vi "电导率电极校准.vi"() -> ()   [LabVIEW 2016, in "斯坦道多参数.lvlib"]
uses:
  <vilib>/Utility/miscctls.llb/LVPointTypeDef.ctl
  <vilib>/Analysis/NI_AALBase.lvlib
panel:
  out "通讯状态":string
  out "盐度":dbl caption="盐度测量值" format="%#.2f"
  out "温度":dbl format="%#.2f"
  out "当前信号值":dbl caption="信号值" format="%#.2f"
  in  "校准停止":bool
  in  "校准启动":bool
  out "波形图表":sgl(graph) caption="历史曲线"
  out "第二点校准值":dbl
  out "第一点校准值":dbl
  in  "校准模式":enum16{"两点校准", "单点校准"}(ring)=enum."单点校准"
  out "提示":string
  out "最小值":sgl format="%#.2f"
  out "最大值":sgl format="%#.2f"
  out "mean":dbl caption="均值" format="%#.2f"
  out "standard deviation":dbl caption="标准差" format="%#.2f"
  out "变异系数":dbl format="%#.6f"
  out "标液2":dbl
  out "标液1":dbl
  out "当前读取值":dbl caption="测量值" format="%#.2f"
  out "电极系数":dbl format="%#.6f"
  out "偏移值补偿":dbl format="%#.2f"
  out "温度补偿系数":dbl caption="温度系数" format="%#.6f"
  # "电导率电极设定"
  # "ppt"
  # "请选择校准模式:"
  # "℃"
  # "uS/cm"
  # "uS/cm"
  # "cm"
  # "-1"
  # "uS/cm"
  # "%"
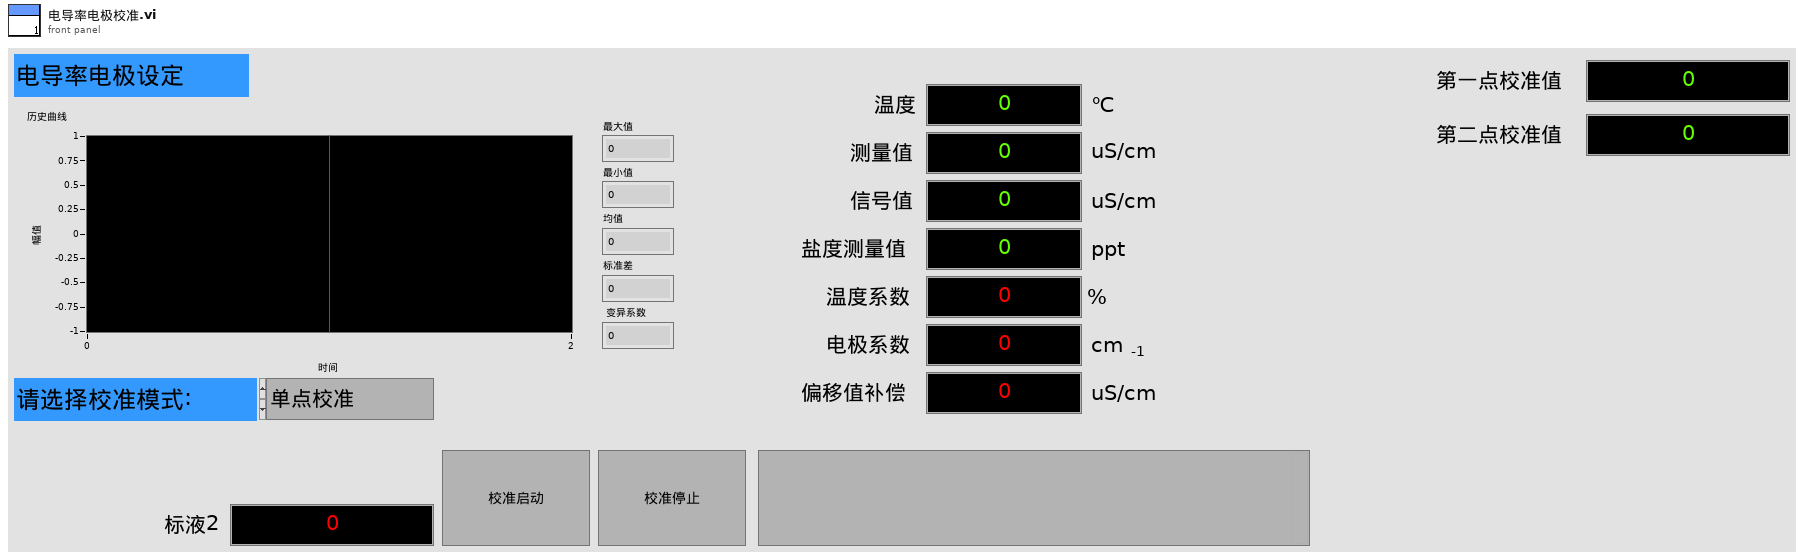
[diagram p1: front panel]
types:
  T1 = typedef "斯坦道多参数.lvlib/校准步骤.ctl" = enum16{"待机", "放置第一点标液", "第一点校准启动", "第一点校准写入", "第一点校准失败", "放置第二点标液", "第二点校准启动", "第二点校准写入", "第二点校准失败", "放置第三点标液", "第三点校准启动", "第三点校准写入", "第三点校准失败", "校准结果写入", "校准结束"}
  T2 = typedef "LVPointTypeDef.ctl" = cluster{"Horizontal":i16, "Vertical":i16}
  T3 = cluster{"电极状态标志":u16, "电极型号标志":u16, "电导率测量值":sgl, "温度测量值":sgl, "电导率信号值":sgl, "温度信号值":sgl, "温度补偿系数":sgl, "电导率偏移修正值":sgl, "温度偏移修正值":sgl, "手动温度补偿值":sgl, "电导率电极零点":sgl, "电导率电极斜率":sgl, "命令滤波设定":u16, "温度模式":enum16{"ATC", "MTC"}, "生产批次":u16, "电极序号":u16, "串口地址":u16, "串口波特率":enum16{"9600", "19200", "115200"}, "串口校验位":enum16{"NONE", "ODD", "EVEN"}, "串口停止位":enum16{"1bit", "2bit"}, "第一点标准值":sgl, "第二点标准值":sgl}
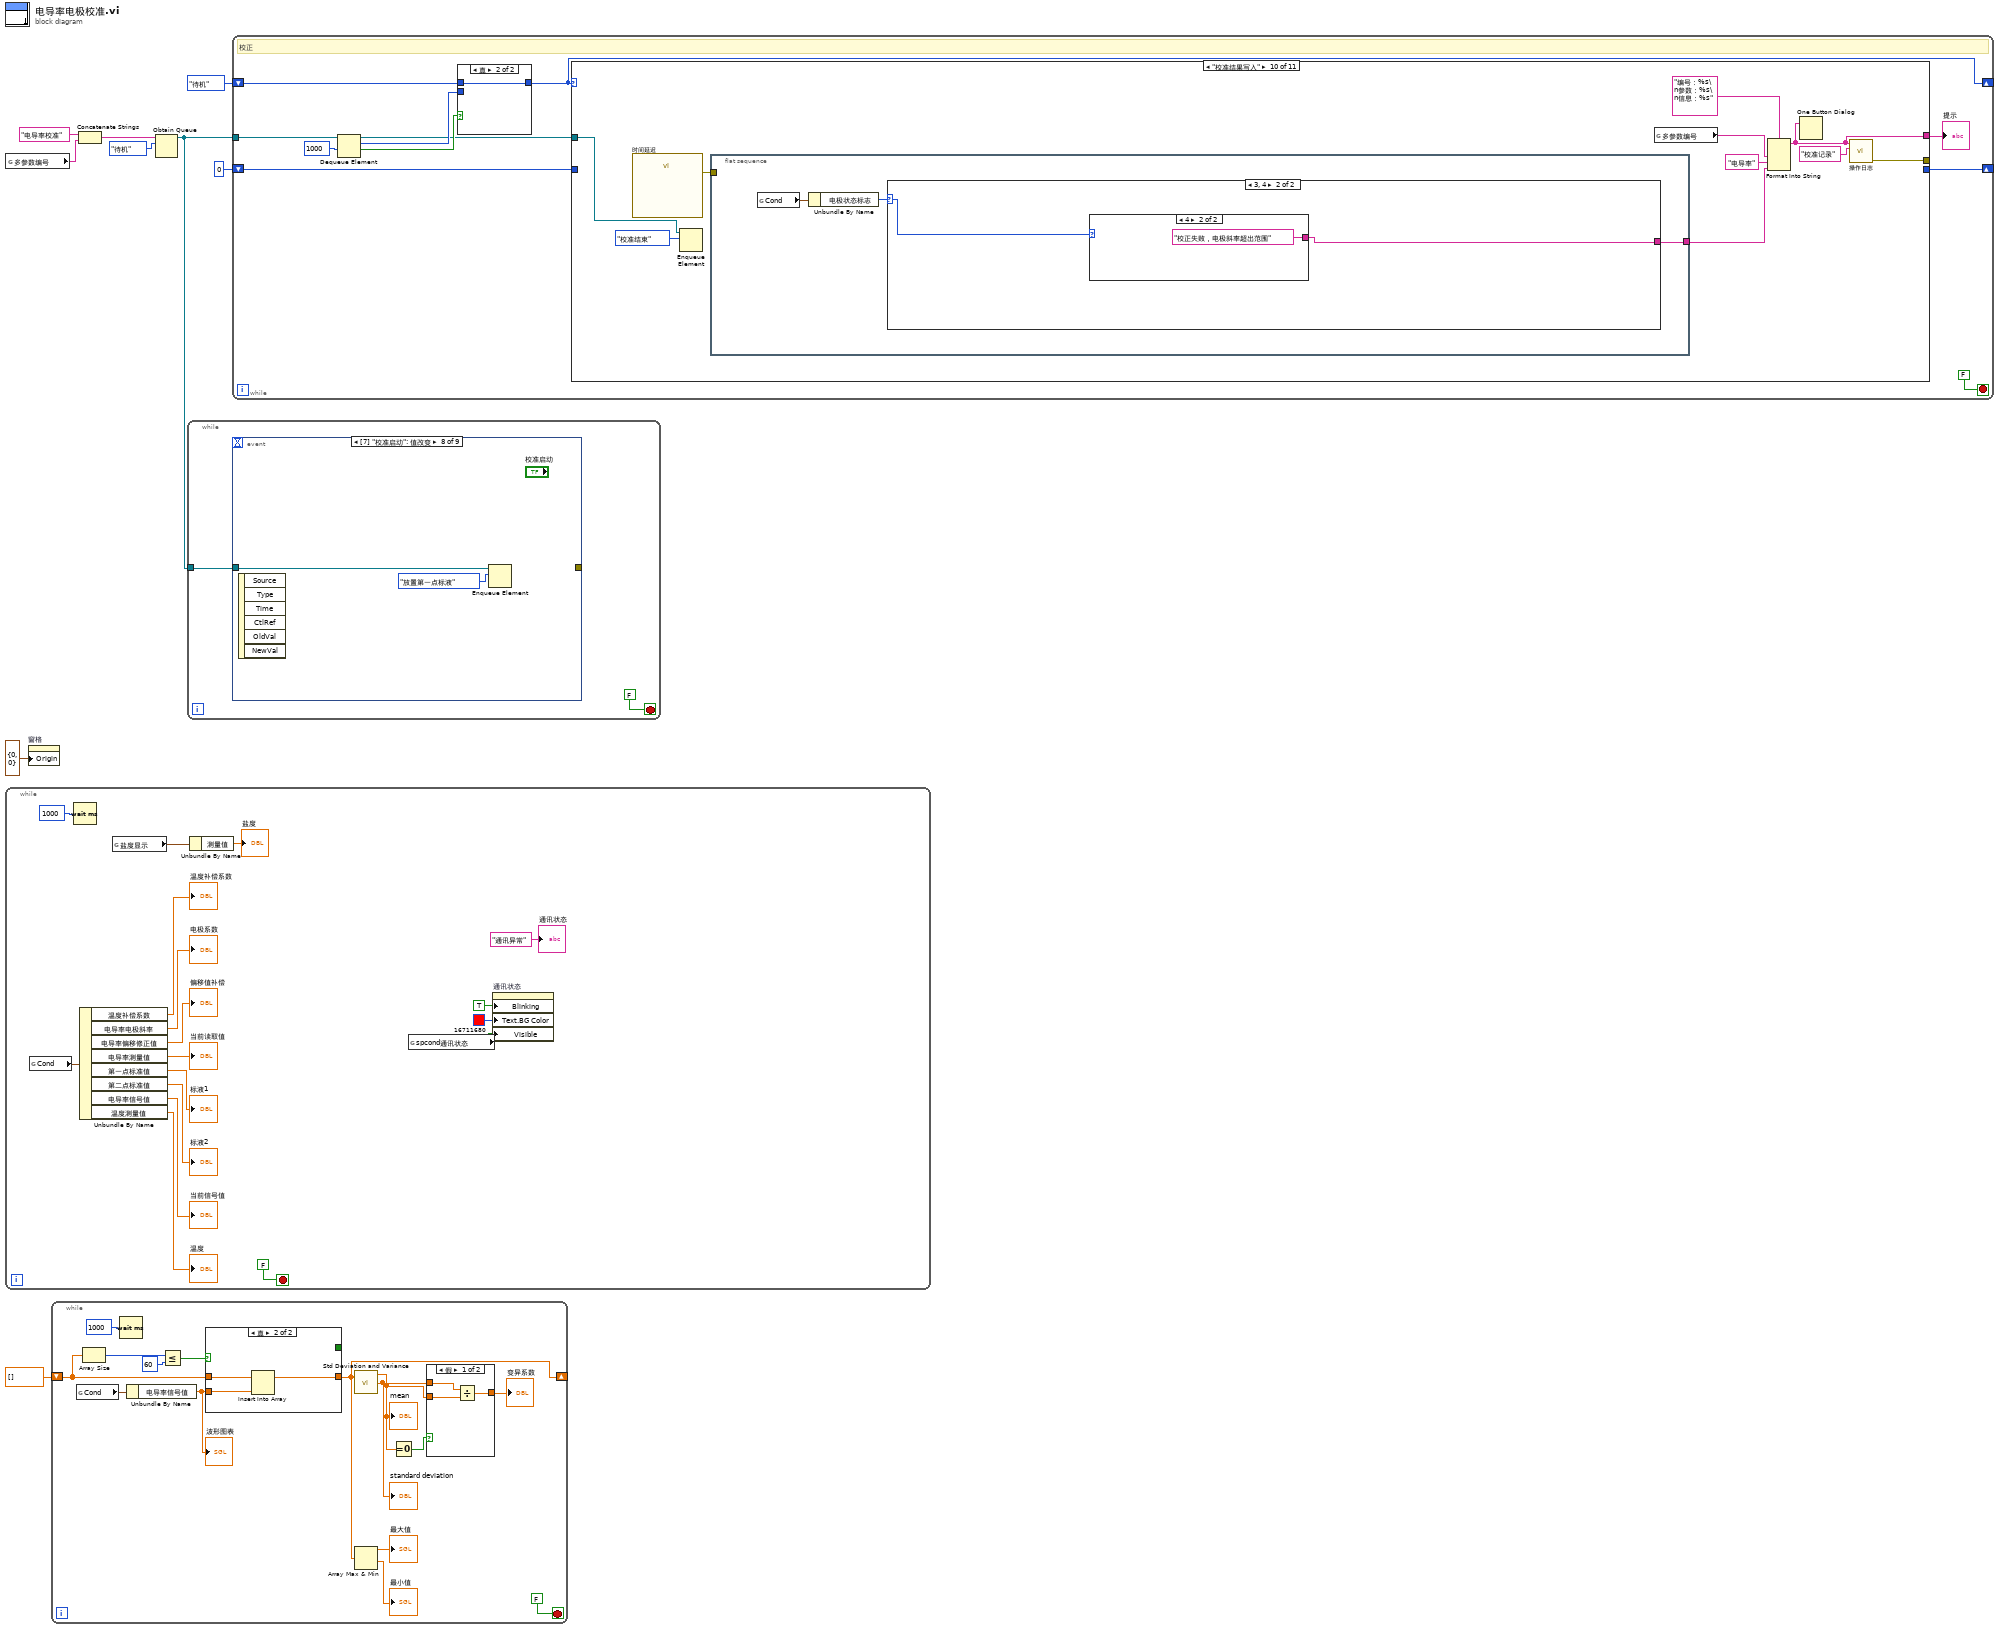
[diagram p0: block diagram]
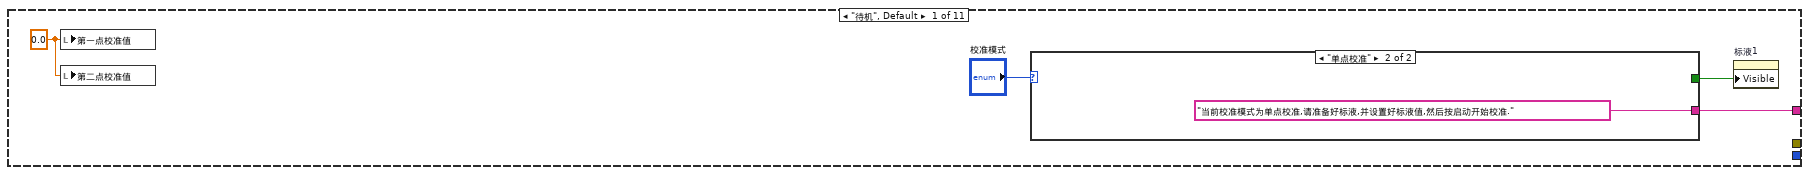
[diagram p3: hidden frame]
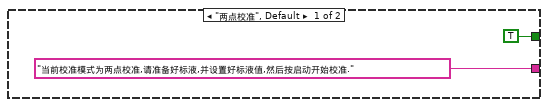
[diagram p4: hidden frame]
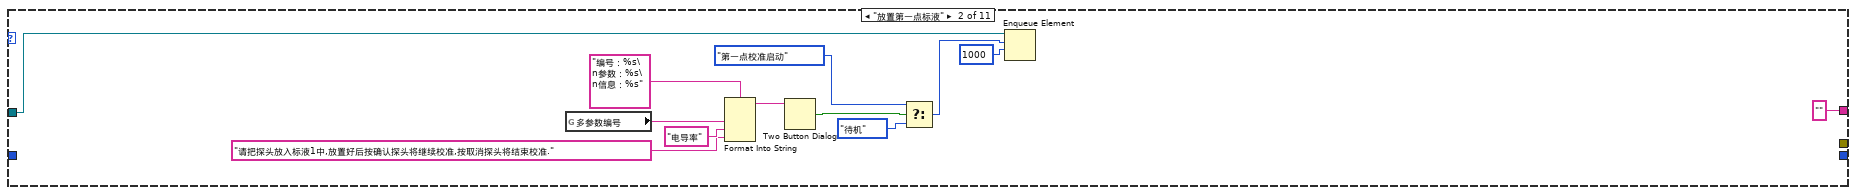
[diagram p5: hidden frame]
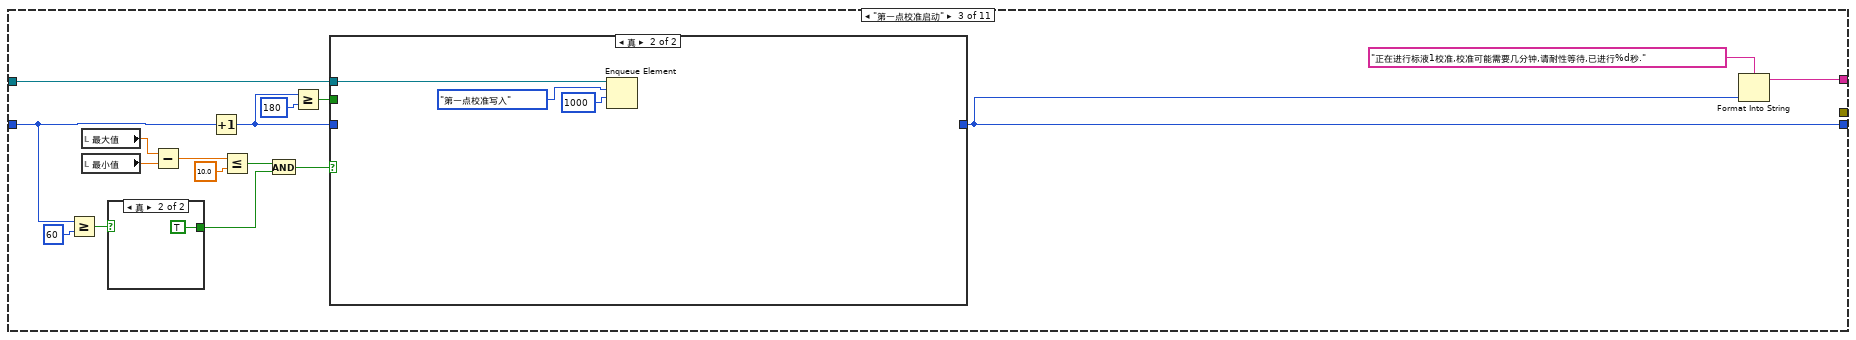
[diagram p6: hidden frame]
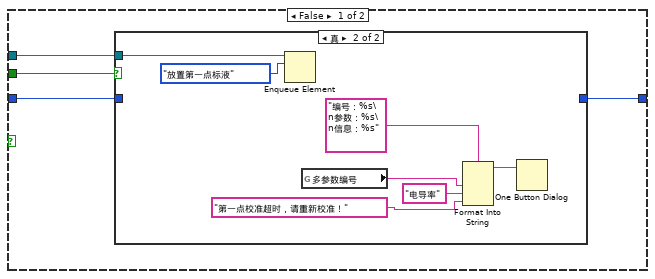
[diagram p7: hidden frame]
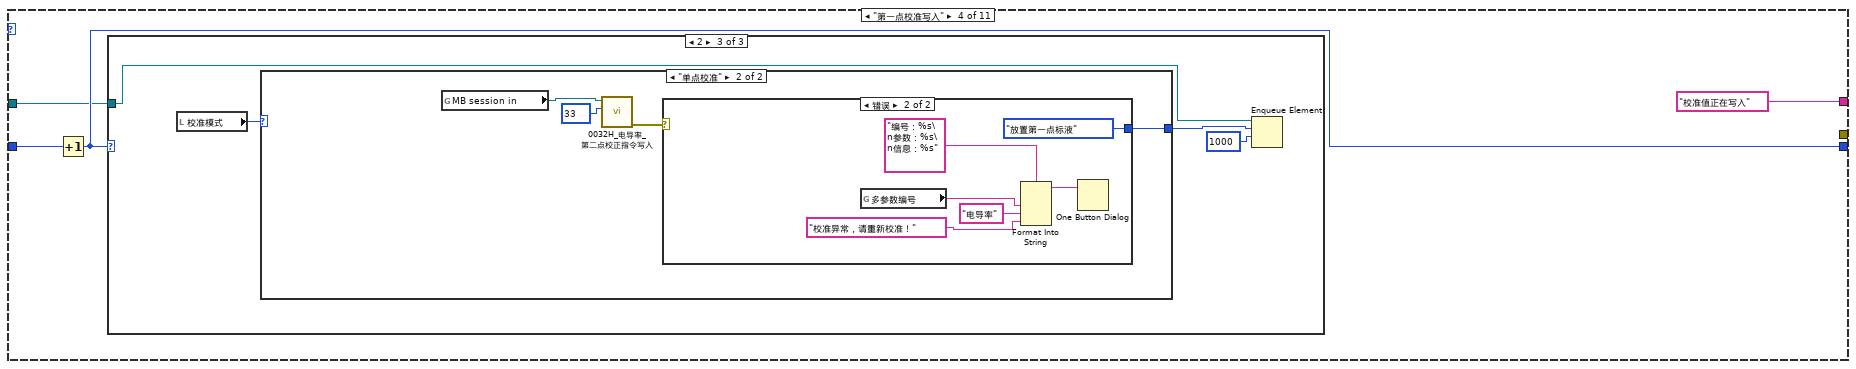
[diagram p10: hidden frame]
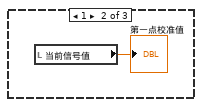
[diagram p12: hidden frame]
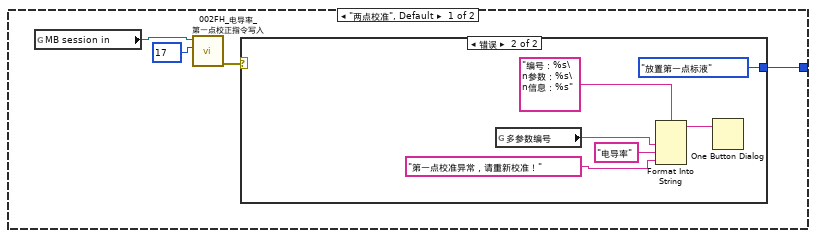
[diagram p13: hidden frame]
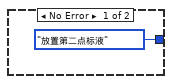
[diagram p14: hidden frame]
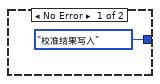
[diagram p15: hidden frame]
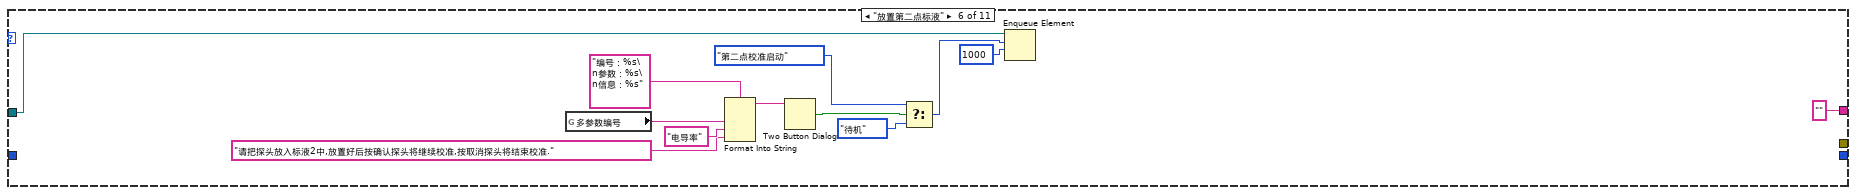
[diagram p17: hidden frame]
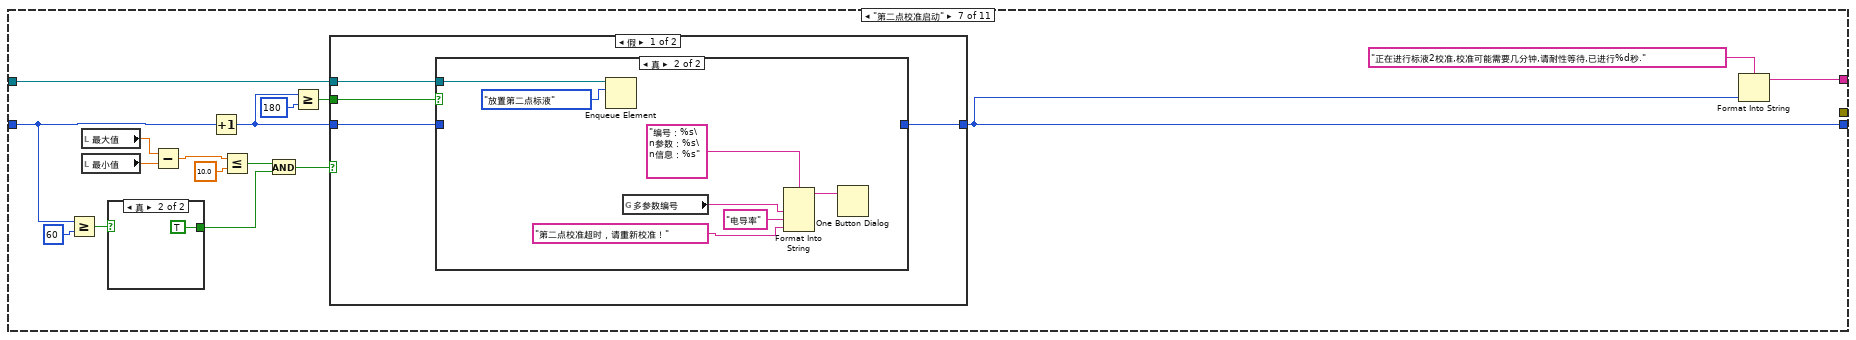
[diagram p18: hidden frame]
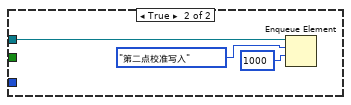
[diagram p20: hidden frame]
diagram:
  n1 = global read "多参数全局变量.vi" "多参数编号"() -> (w1:string)
  n2 = while {
    stop <- FALSE stop-if-true
    n3 = global read "国弘过程全局变量.vi" "Cond"() -> (w24:T3)
    n4 = Wait (ms)(milliseconds to wait=u32 1000 ("等待时间（毫秒）")) -> ()  [unwired: 1 out]
    n5 = Unbundle By Name(w24) -> ("温度补偿系数"=→"温度补偿系数":sgl, "电导率电极斜率"=→"电极系数":sgl, "电导率偏移修正值"=→"偏移值补偿":sgl, "电导率测量值"=→"当前读取值":sgl, "第一点标准值"=→"标液1":sgl, "第二点标准值"=→"标液2":sgl, "电导率信号值"=→"当前信号值":sgl, "温度测量值"=→"温度":sgl)
    n6 = global read "多参数全局变量.vi" "盐度显示"() -> (w15:cluster{"温度测量值":sgl, "测量值":sgl, "温度偏移修正值":sgl})
    n7 = Unbundle By Name(w15) -> ("测量值"=→"盐度":sgl)
    n8 = global read "多参数全局变量.vi" "spcond通讯状态"() -> (w10:bool)
    n9 = property on="通讯状态" class="Str"("Blinking"=TRUE ("闪烁"), "Text.BG Color"=u32 16711680, "Visible"=w10) -> ()  [unwired: 2 in, 2 out]
    "通讯状态" <- "通讯异常" ("当前串口")
  }
  n10 = property on="窗格" class="Pane"("Origin"=T2 {"Horizontal"=0, "Vertical"=0} ("原点")) -> ()  [unwired: 2 in, 2 out]
  n11 = while {
    shift-right: [w30] -> _
    shift-left: sgl[] [] -> [w37]
    stop <- FALSE stop-if-true
    n12 = global read "国弘过程全局变量.vi" "Cond"() -> (w31:T3)
    n13 = Array Size(array=w37) -> (size(s)=w39:i32)
    n14 = Wait (ms)(milliseconds to wait=u32 1000 ("等待时间（毫秒）")) -> ()  [unwired: 1 out]
    n15 = Unbundle By Name(w31) -> ("电导率信号值"=w27:sgl)
    "波形图表" <- w27
    n16 = Less Or Equal?(x=w39, y=60) -> (x <= y?=w38:bool)
    n17 = case shown="真" w38 {
      tunnel: w37 -> [w50 w53]
      tunnel: w27 -> [w48 w52]
      tunnel: [w46 w51] -> w30
      tunnel: [TRUE _] -> _
      frame False {
        n18 = Replace Array Subset(array=w50, new element=w48) -> (w49:sgl[])  [unwired: 1 in]
        n19 = Rotate 1D Array(1:w49, 2:-1 ("n")) -> (0:w46:sgl[])
      }
      frame True {
        n20 = Insert Into Array(array=w53, new element=w52) -> (w51:sgl[])  [unwired: 1 in]
      }
    }
    n21 = call <vilib>:"Std Deviation and Variance.vi"("X"=w30) -> ("mean"=w35:dbl, "standard deviation"=w34:dbl)  [unwired: 1 in, 1 out]
    "mean" <- w35
    "standard deviation" <- w34
    n22 = Array Max & Min(array=w30) -> (max value=→"最大值":sgl, min value=→"最小值":sgl)  [unwired: 2 out]
    n23 = Equal To 0?(x=w35) -> (x = 0?=w36:bool)
    n24 = case shown="假" w36 {
      tunnel: w34 -> [w44 _]
      tunnel: [w43 _] -> w33
      tunnel: w35 -> [w42 _]
      frame False {
        n25 = Divide(x=w44, y=w42) -> (x/y=w43:dbl)
      }
      frame True {
      }
    }
    "变异系数" <- w33
  }
  n26 = Concatenate Strings("电导率校准" ("名称（未命名）"), w1) -> (w2:string)
  n27 = Obtain Queue(name (unnamed)=w2, element data type=校准步骤."待机" ("枚举")) -> (queue out=w3:refnum<queue>)  [unwired: 3 in, 2 out]
  n28 = while {
    tunnel: w3 -> [w54]
    stop <- FALSE stop-if-true
    n29 = event shown="[7] \"校准启动\": 值改变" {
      selector: _ -> [_ _ _ _ _ _ _ _ _]
      dyn-events: _ -> [_ _ _ _ _ _ _ _ _]
      timeout: _ -> [_ _ _ _ _ _ _ _ _]
      tunnel: [_ _ w61 w64 w67 w71 w74 _ _] -> _
      tunnel: w54 -> [_ _ _ _ _ _ _ w76 w77]
      event Timeout {
        n30 = event-data() -> ()  [unwired: 1 in, 3 out]
      }
      event "偏移值补偿", "标液2", "电极系数", "温度补偿系数": Mouse Down {
        n31 = event-data() -> ("CtlRef"=w56:refnum<vi>)  [unwired: 1 in, 7 out]
        n32 = property class="DigNum (严格)"(reference=w56) -> (reference out=w57:refnum<vi>, "Value"=w58:dbl)  [unwired: 1 in, 1 out]
        n33 = call "数字键盘.vi"("OldNumber"=w58) -> ("NewNumber"=w59:dbl)  [unwired: 1 in]
        n34 = property class="DigNum (严格)"(reference=w57, "Val(Sgnl)"=w59) -> ()  [unwired: 1 in, 2 out]
      }
      event "温度补偿系数": Value Change {
        n35 = event-data() -> ("NewVal"=w62:dbl)  [unwired: 1 in, 5 out]
        n36 = global read "多参数全局变量.vi" "MB session in"() -> (w60:refnum<class "MB_Master.lvclass">)
        n37 = call "000AH_电导率_温度补偿系数写入.vi"("数值"=w62, "MB session in"=w60) -> ("error out"=w61:errorcluster)  [unwired: 8 in, 1 out]
      }
      event "偏移值补偿": Value Change {
        n38 = event-data() -> ("NewVal"=w65:dbl)  [unwired: 1 in, 5 out]
        n39 = global read "多参数全局变量.vi" "MB session in"() -> (w63:refnum<class "MB_Master.lvclass">)
        n40 = call "000CH_电导率_电导率偏移修正值写入.vi"("数值"=w65, "MB session in"=w63) -> ("error out"=w64:errorcluster)  [unwired: 8 in, 1 out]
      }
      event "标液1": Value Change {
        n41 = event-data() -> ("NewVal"=w68:dbl)  [unwired: 1 in, 5 out]
        n42 = global read "多参数全局变量.vi" "MB session in"() -> (w66:refnum<class "MB_Master.lvclass">)
        n43 = call "0030H_电导率_第一点标准值写入.vi"("数值"=w68, "MB session in"=w66) -> ("error out"=w67:errorcluster)  [unwired: 8 in, 1 out]
      }
      event "标液2": Value Change {
        n44 = event-data() -> ("NewVal"=w70:dbl)  [unwired: 1 in, 5 out]
        n45 = global read "多参数全局变量.vi" "MB session in"() -> (w69:refnum<class "MB_Master.lvclass">)
        n46 = call "0033H_电导率_第二点标准值写入.vi"("数值"=w70, "MB session in"=w69) -> ("error out"=w71:errorcluster)  [unwired: 8 in, 1 out]
      }
      event "电极系数": Value Change {
        n47 = event-data() -> ("NewVal"=w73:dbl)  [unwired: 1 in, 5 out]
        n48 = global read "多参数全局变量.vi" "MB session in"() -> (w72:refnum<class "MB_Master.lvclass">)
        n49 = call "0014H_电导率_电极系数写入.vi"("数值"=w73, "MB session in"=w72) -> ("error out"=w74:errorcluster)  [unwired: 8 in, 1 out]
      }
      event "校准启动": Value Change {
        n50 = event-data() -> ()  [unwired: 1 in, 6 out]
        n51 = Enqueue Element(queue=w76, element=校准步骤."放置第一点标液" ("元素")) -> ()  [unwired: 2 in, 3 out]
      }
      event "校准停止": Value Change {
        n52 = event-data() -> ()  [unwired: 1 in, 6 out]
        n53 = Flush Queue(queue=w77) -> (queue out=w78:refnum<queue>)  [unwired: 1 in, 2 out]
        n54 = Enqueue Element(queue=w78, element=校准步骤."待机" ("元素"), timeout in ms (-1)=1000 ("超时毫秒(-1)")) -> ()  [unwired: 1 in, 3 out]
      }
    }
  }
  n55 = while "While循环" {
    shift-right: [w82] -> _
    shift-left: 校准步骤."待机" ("枚举") -> [w83]
    shift-right: [w89] -> _
    shift-left: 0 -> [w90]
    tunnel: w3 -> [w87]
    stop <- FALSE stop-if-true
    # "校正"
    n56 = Dequeue Element(queue=w87, timeout in ms (-1)=1000 ("超时毫秒(-1)")) -> (queue out=w81:refnum<queue>, element=w84:T1, timed out?=w85:bool)  [unwired: 1 in, 1 out]
    n57 = case shown="真" w85 {
      tunnel: w84 -> [w92 _]
      tunnel: [w92 w93] -> w82
      tunnel: w83 -> [_ w93]
      frame False {
      }
      frame True {
      }
    }
    n58 = case shown="\"校准结果写入\"" w82 {
      tunnel: [w97 "" ("提示") w128 "校准值正在写入" ("提示") _ "" ("提示") w204 "校准值正在写入" ("提示") _ w243 w269] -> w88
      tunnel: w90 -> [_ _ w122 w148 _ _ w198 w224 _ _ _]
      tunnel: [_ _ w113 w147 _ _ w189 w223 _ _ _] -> w89
      tunnel: w81 -> [_ w112 w116 w146 _ w188 w192 w222 _ w249 _]
      tunnel: [_ _ _ _ _ _ _ _ _ w247 _] -> _
      frame "待机", Default {
        w94 = 0.0 ("第一点校准值")
        n59 = local write "第一点校准值"(w94) -> ()
        n60 = local write "第二点校准值"(w94) -> ()
        n61 = case shown="\"单点校准\"" "校准模式" {
          tunnel: ["当前校准模式为两点校准,请准备好标液,并设置好标液值,然后按启动开始校准." ("提示") "当前校准模式为单点校准,请准备好标液,并设置好标液值,然后按启动开始校准." ("提示")] -> w97
          tunnel: [TRUE ("可见") _] -> w96
          frame "两点校准", Default {
          }
          frame "单点校准" {
          }
        }
        n62 = property on="标液1" class="DigNum (严格)"("Visible"=w96) -> ()  [unwired: 2 in, 2 out]
      }
      frame "放置第一点标液" {
        n63 = global read "多参数全局变量.vi" "多参数编号"() -> (w104:string)
        n64 = Format Into String(format string="编号：%s\n参数：%s\n信息：%s" ("格式字符串"), w104, "电导率" ("输入 2"), "请把探头放入标液1中,放置好后按确认探头将继续校准,按取消探头将结束校准." ("消息")) -> (resulting string=w101:string)  [unwired: 2 in, 1 out]
        n65 = Two Button Dialog(message=w101) -> (T button?=w110:bool)  [unwired: 2 in]
        n66 = Select(t=校准步骤."第一点校准启动" ("元素"), s=w110, f=校准步骤."待机" ("元素")) -> (s? t:f=w107:T1)
        n67 = Enqueue Element(queue=w112, element=w107, timeout in ms (-1)=1000 ("超时毫秒(-1)")) -> ()  [unwired: 1 in, 3 out]
      }
      frame "第一点校准启动" {
        n68 = Greater Or Equal?(x=w122, y=60) -> (x >= y?=w123:bool)
        n69 = local read "最大值"() -> (w119:sgl)
        n70 = local read "最小值"() -> (w120:sgl)
        n71 = case shown="真" w123 {
          tunnel: [_ TRUE] -> w121
          frame False {
          }
          frame True {
          }
        }
        n72 = Subtract(x=w119, y=w120) -> (x-y=w118:sgl)
        n73 = Increment(x=w122) -> (x+1=w114:i32)
        n74 = Less Or Equal?(x=w118, y=10.0) -> (x <= y?=w126:bool)
        n75 = And(x=w126, y=w121) -> (x .and. y?=w117:bool)
        n76 = Greater Or Equal?(x=w114, y=180) -> (x >= y?=w115:bool)
        n77 = case shown="真" w117 {
          tunnel: w116 -> [w132 w144]
          tunnel: w115 -> [w133 _]
          tunnel: w114 -> [w131 _]
          tunnel: [w130 _] -> w113
          frame False {
            n78 = case shown="真" w133 {
              tunnel: w132 -> [_ w141]
              tunnel: w131 -> [w134 _]
              tunnel: [w134 _] -> w130
              frame False {
              }
              frame True {
                n79 = Enqueue Element(queue=w141, element=校准步骤."放置第一点标液" ("元素")) -> ()  [unwired: 2 in, 3 out]
                n80 = global read "多参数全局变量.vi" "多参数编号"() -> (w138:string)
                n81 = Format Into String(format string="编号：%s\n参数：%s\n信息：%s" ("格式字符串"), w138, "电导率" ("输入 2"), "第一点校准超时，请重新校准！" ("error source (\" \")")) -> (resulting string=w136:string)  [unwired: 2 in, 1 out]
                n82 = One Button Dialog(message=w136) -> ()  [unwired: 1 in, 1 out]
              }
            }
          }
          frame True {
            n83 = Enqueue Element(queue=w144, element=校准步骤."第一点校准写入" ("元素"), timeout in ms (-1)=1000 ("超时毫秒(-1)")) -> ()  [unwired: 1 in, 3 out]
          }
        }
        n84 = Format Into String(format string="正在进行标液1校准,校准可能需要几分钟,请耐性等待,已进行%d秒." ("格式字符串"), w113) -> (resulting string=w128:string)  [unwired: 2 in, 1 out]
      }
      frame "第一点校准写入" {
        n85 = Increment(x=w148) -> (x+1=w147:i32)
        n86 = case shown="2" w147 {
          tunnel: w146 -> [_ _ w154]
          frame 0, Default {
          }
          frame 1 {
            n87 = local read "当前信号值"() -> (→"第一点校准值":dbl)
          }
          frame 2 {
            n88 = local read "校准模式"() -> (w153:enum16{"两点校准", "单点校准"})
            n89 = case shown="\"单点校准\"" w153 {
              tunnel: [w158 w166] -> w152
              frame "两点校准", Default {
                n90 = global read "多参数全局变量.vi" "MB session in"() -> (w156:refnum<class "MB_Master.lvclass">)
                n91 = call "002FH_电导率_第一点校正指令写入.vi"("数值"=u16 17, "MB session in"=w156) -> ("error out"=w157:errorcluster)  [unwired: 8 in, 1 out]
                n92 = case shown="错误" w157 {
                  tunnel: [校准步骤."放置第二点标液" ("元素") 校准步骤."放置第一点标液" ("元素")] -> w158
                  frame No Error {
                  }
                  frame Error {
                    n93 = global read "多参数全局变量.vi" "多参数编号"() -> (w162:string)
                    n94 = Format Into String(format string="编号：%s\n参数：%s\n信息：%s" ("格式字符串"), w162, "电导率" ("输入 2"), "第一点校准异常，请重新校准！" ("error source (\" \")")) -> (resulting string=w160:string)  [unwired: 2 in, 1 out]
                    n95 = One Button Dialog(message=w160) -> ()  [unwired: 1 in, 1 out]
                  }
                }
              }
              frame "单点校准" {
                n96 = global read "多参数全局变量.vi" "MB session in"() -> (w169:refnum<class "MB_Master.lvclass">)
                n97 = call "0032H_电导率_第二点校正指令写入.vi"("数值"=u16 33, "MB session in"=w169) -> ("error out"=w167:errorcluster)  [unwired: 8 in, 1 out]
                n98 = case shown="错误" w167 {
                  tunnel: [校准步骤."校准结果写入" ("元素") 校准步骤."放置第一点标液" ("元素")] -> w166
                  frame No Error {
                  }
                  frame Error {
                    n99 = global read "多参数全局变量.vi" "多参数编号"() -> (w174:string)
                    n100 = Format Into String(format string="编号：%s\n参数：%s\n信息：%s" ("格式字符串"), w174, "电导率" ("输入 2"), "校准异常，请重新校准！" ("error source (\" \")")) -> (resulting string=w173:string)  [unwired: 2 in, 1 out]
                    n101 = One Button Dialog(message=w173) -> ()  [unwired: 1 in, 1 out]
                  }
                }
              }
            }
            n102 = Enqueue Element(queue=w154, element=w152, timeout in ms (-1)=1000 ("超时毫秒(-1)")) -> ()  [unwired: 1 in, 3 out]
          }
        }
      }
      frame "第一点校准失败" {
      }
      frame "放置第二点标液" {
        n103 = global read "多参数全局变量.vi" "多参数编号"() -> (w180:string)
        n104 = Format Into String(format string="编号：%s\n参数：%s\n信息：%s" ("格式字符串"), w180, "电导率" ("输入 2"), "请把探头放入标液2中,放置好后按确认探头将继续校准,按取消探头将结束校准." ("消息")) -> (resulting string=w177:string)  [unwired: 2 in, 1 out]
        n105 = Two Button Dialog(message=w177) -> (T button?=w186:bool)  [unwired: 2 in]
        n106 = Select(t=校准步骤."第二点校准启动" ("元素"), s=w186, f=校准步骤."待机" ("元素")) -> (s? t:f=w183:T1)
        n107 = Enqueue Element(queue=w188, element=w183, timeout in ms (-1)=1000 ("超时毫秒(-1)")) -> ()  [unwired: 1 in, 3 out]
      }
      frame "第二点校准启动" {
        n108 = Greater Or Equal?(x=w198, y=60) -> (x >= y?=w199:bool)
        n109 = local read "最大值"() -> (w195:sgl)
        n110 = local read "最小值"() -> (w196:sgl)
        n111 = case shown="真" w199 {
          tunnel: [_ TRUE] -> w197
          frame False {
          }
          frame True {
          }
        }
        n112 = Subtract(x=w195, y=w196) -> (x-y=w194:sgl)
        n113 = Increment(x=w198) -> (x+1=w190:i32)
        n114 = Less Or Equal?(x=w194, y=10.0) -> (x <= y?=w202:bool)
        n115 = And(x=w202, y=w197) -> (x .and. y?=w193:bool)
        n116 = Greater Or Equal?(x=w190, y=180) -> (x >= y?=w191:bool)
        n117 = case shown="假" w193 {
          tunnel: w192 -> [w208 w220]
          tunnel: w191 -> [w209 _]
          tunnel: w190 -> [w207 _]
          tunnel: [w206 _] -> w189
          frame False {
            n118 = case shown="真" w209 {
              tunnel: w208 -> [_ w217]
              tunnel: w207 -> [w210 _]
              tunnel: [w210 _] -> w206
              frame False {
              }
              frame True {
                n119 = Enqueue Element(queue=w217, element=校准步骤."放置第二点标液" ("元素")) -> ()  [unwired: 2 in, 3 out]
                n120 = global read "多参数全局变量.vi" "多参数编号"() -> (w214:string)
                n121 = Format Into String(format string="编号：%s\n参数：%s\n信息：%s" ("格式字符串"), w214, "电导率" ("输入 2"), "第二点校准超时，请重新校准！" ("error source (\" \")")) -> (resulting string=w212:string)  [unwired: 2 in, 1 out]
                n122 = One Button Dialog(message=w212) -> ()  [unwired: 1 in, 1 out]
              }
            }
          }
          frame True {
            n123 = Enqueue Element(queue=w220, element=校准步骤."第二点校准写入" ("元素"), timeout in ms (-1)=1000 ("超时毫秒(-1)")) -> ()  [unwired: 1 in, 3 out]
          }
        }
        n124 = Format Into String(format string="正在进行标液2校准,校准可能需要几分钟,请耐性等待,已进行%d秒." ("格式字符串"), w189) -> (resulting string=w204:string)  [unwired: 2 in, 1 out]
      }
      frame "第二点校准写入" {
        n125 = Increment(x=w224) -> (x+1=w223:i32)
        n126 = case shown="0, 默认" w223 {
          tunnel: w222 -> [_ _ w232]
          frame 0, Default {
          }
          frame 1 {
            n127 = local read "当前信号值"() -> (→"第二点校准值":dbl)
          }
          frame 2 {
            n128 = global read "多参数全局变量.vi" "MB session in"() -> (w229:refnum<class "MB_Master.lvclass">)
            n129 = call "0032H_电导率_第二点校正指令写入.vi"("数值"=u16 33, "MB session in"=w229) -> ("error out"=w227:errorcluster)  [unwired: 8 in, 1 out]
            n130 = case shown="错误" w227 {
              tunnel: [校准步骤."校准结果写入" ("元素") 校准步骤."放置第二点标液" ("元素")] -> w230
              frame No Error {
              }
              frame Error {
                n131 = global read "多参数全局变量.vi" "多参数编号"() -> (w236:string)
                n132 = Format Into String(format string="编号：%s\n参数：%s\n信息：%s" ("格式字符串"), w236, "电导率" ("输入 2"), "第二点校准异常，请重新校准！" ("error source (\" \")")) -> (resulting string=w234:string)  [unwired: 2 in, 1 out]
                n133 = One Button Dialog(message=w234) -> ()  [unwired: 1 in, 1 out]
              }
            }
            n134 = Enqueue Element(queue=w232, element=w230, timeout in ms (-1)=1000 ("超时毫秒(-1)")) -> ()  [unwired: 1 in, 3 out]
          }
        }
      }
      frame "第二点校准失败" {
      }
      frame "校准结果写入" {
        n135 = call "时间延迟"() -> ("error out"=w240:errorcluster)  [unwired: 11 in]
        n136 = Enqueue Element(queue=w249, element=校准步骤."校准结束" ("元素")) -> ()  [unwired: 2 in, 3 out]
        n137 = flat-sequence {
          tunnel: [w250] -> w242
          tunnel: w240 -> [_]
          frame #0 {
            n138 = global read "国弘过程全局变量.vi" "Cond"() -> (w252:T3)
            n139 = Unbundle By Name(w252) -> ("电极状态标志"=w251:u16)
            n140 = case shown="3, 4" w251 {
              selector: w251 -> [_ w266]
              tunnel: [w254 w265] -> w250
              frame 0, Default {
                n141 = local read "校准模式"() -> (w253:enum16{"两点校准", "单点校准"})
                n142 = case shown="\"两点校准\", 默认" w253 {
                  tunnel: [w258 w263] -> w254
                  frame "两点校准", Default {
                    n143 = local read "第一点校准值"() -> (w259:dbl)
                    n144 = local read "第二点校准值"() -> (w256:dbl)
                    n145 = local read "标液1"() -> (w260:dbl)
                    n146 = local read "标液2"() -> (w255:dbl)
                    n147 = Format Into String(format string="校准结果：第一点校准值=%f，第一点标准值=%f,第二点校准值=%f，第二点标准值=%f." ("提示"), w259, w260, w256, w255) -> (resulting string=w258:string)  [unwired: 2 in, 1 out]
                  }
                  frame "单点校准" {
                    n148 = local read "第一点校准值"() -> (w264:dbl)
                    n149 = local read "标液2"() -> (w261:dbl)
                    n150 = Format Into String(format string="校准结果：校准值=%f，标准值=%f。" ("提示"), w264, w261) -> (resulting string=w263:string)  [unwired: 2 in, 1 out]
                  }
                }
              }
              frame 3, 4 {
                n151 = case shown="4" w266 {
                  tunnel: ["校正失败，电极零点超出范围" "校正失败，电极斜率超出范围"] -> w265
                  frame 3, Default {
                  }
                  frame 4 {
                  }
                }
              }
            }
          }
        }
        n152 = global read "多参数全局变量.vi" "多参数编号"() -> (w245:string)
        n153 = Format Into String(format string="编号：%s\n参数：%s\n信息：%s" ("格式字符串"), w245, "电导率" ("输入 2"), w242) -> (resulting string=w243:string)  [unwired: 2 in, 1 out]
        n154 = One Button Dialog(message=w243) -> ()  [unwired: 1 in, 1 out]
        n155 = call "操作日志.vi"("table"="校准记录", "日志信息"=w243) -> ("error out"=w247:errorcluster)  [unwired: 9 in]
      }
      frame "校准结束" {
        n156 = local read "提示"() -> (w269:string)
      }
    }
    "提示" <- w88
  }
